vi "simple build.vi"() -> ()   [LabVIEW 2016]
uses:
  <vilib>/AppBuilder/AB_API/PPL/NI_AB_API_PPL.lvclass
panel:
  out "Array":string[](array[string])
  out "error out":errorcluster
  in  "Path":path
  in  "Build specification name":string
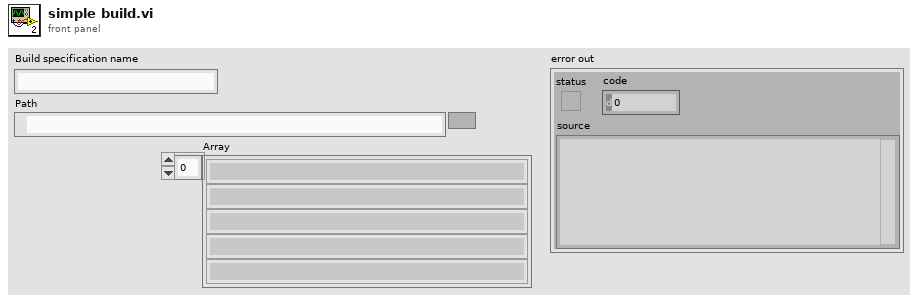
[diagram p1: front panel]
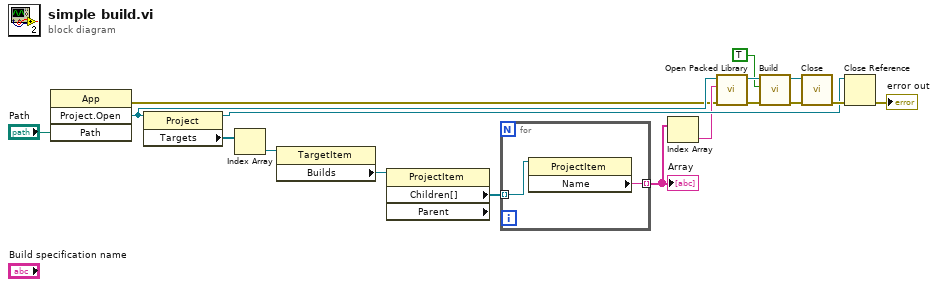
[diagram p0: block diagram]
diagram:
  n1 = invoke class="App" method="Project.Open"("Path"="Path") -> (error out=w4:errorcluster, "Project:Open"=w6:refnum<vi>)  [unwired: 3 in, 2 out]
  n2 = property class="Project"(reference=w6) -> (reference out=w8:refnum<vi>, "Targets"=w14:refnum<vi>[])  [unwired: 1 in, 1 out]
  n3 = Index Array(array=w14) -> (element=w13:refnum<vi>)  [unwired: 1 in]
  n4 = property class="TargetItem"(reference=w13) -> ("Builds"=w12:refnum<vi>)  [unwired: 1 in, 2 out]
  n5 = property class="ProjectItem" props=["Children[]", "Parent"](reference=w12) -> ("Children[]"=w11:refnum<vi>[])  [unwired: 1 in, 3 out]
  n6 = for {
    tunnel: w11 -> [w19] mode=indexing
    tunnel: [w18] -> w10 mode=indexing
    n7 = property class="ProjectItem"(reference=w19) -> ("Name"=w18:string)  [unwired: 1 in, 2 out]
  }
  "Array" <- w10
  n8 = Index Array(array=w10) -> (element=w5:string)  [unwired: 1 in]
  n9 = call <vilib>:"Open Packed Library.vi"("error in (no error)"=w4, "Build specification name"=w5, "Project Refnum"=w6) -> ("error out"=w2:errorcluster, "PPL out"=w3:refnum<class "NI_AB_API_PPL.lvclass">)  [unwired: 7 in]
  n10 = call-dynamic "Build.vi"("error in (no error)"=w2, "collect dependencies? (F)"=TRUE, "PPL in"=w3) -> ("error out"=w17:errorcluster, "PPL out"=w16:refnum<class "NI_AB_API_PPL.lvclass">)  [unwired: 5 in, 2 out]
  n11 = call-dynamic "Close.vi"("error in (no error)"=w17, "DLL in"=w16) -> ("error out"=w9:errorcluster)  [unwired: 9 in]
  n12 = Close Reference(reference=w8, error in (no error)=w9) -> (error out=→"error out":errorcluster)
